vi "EraseRawDataChannels.vi"(7 "error in":errorcluster, 9 "File Limit Size":i64, 10 "TDMS file path in":path) -> (0 "error out":errorcluster, 2 "num chans":i32, 3 "TDMS file path out":path)   [LabVIEW 2012]
uses:
  <vilib>/Platform/storage/lvStorage.llb/_openStorageWithRootAutoDetect.vi
  <vilib>/Platform/storage/lvStorage.llb/xStorage/xStorageSupp/ErrorOut.vi
  <vilib>/Platform/storage/Storage.llb/__loadPropString.vi
  <vilib>/Platform/storage/Storage.llb/__loadPropTime.vi
  <vilib>/Platform/storage/Storage.llb/__loadPropRefList.vi
  <vilib>/Platform/storage/lvStorage.llb/_loadDDT.vi
  <vilib>/Platform/storage/lvStorage.llb/Delete Channel.vi
  <vilib>/Platform/storage/Storage.llb/Get Object Info.vi
  <vilib>/Platform/storage/Storage.llb/__closeStorageFromObject.vi
  <vilib>/ErrorRing/Error Ring.xnode
  <vilib>/Platform/storage/lvStorage.llb/xStorage/Open Data Storage/Open Data Storage.xnode
  <vilib>/Platform/storage/lvStorage.llb/xStorage/Get Properties/Get Properties.xnode
  <vilib>/Platform/storage/lvStorage.llb/xStorage/Close Data Storage/Close Data Storage.xnode
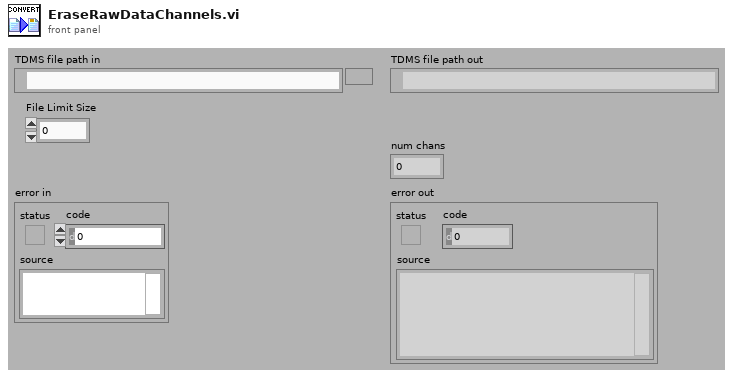
[diagram p1: front panel]
types:
  T1 = enum16{"open", "open or create", "create or replace", "create", "open (read only)"}
  T2 = enum16{"open", "open or create", "create or replace", "create", "open (read-only)"}
  T3 = enum16{"UPDATE", "READ", "QUERY", "CREATE CHILD", "CREATE", "CONNECT", "DISCONNECT"}
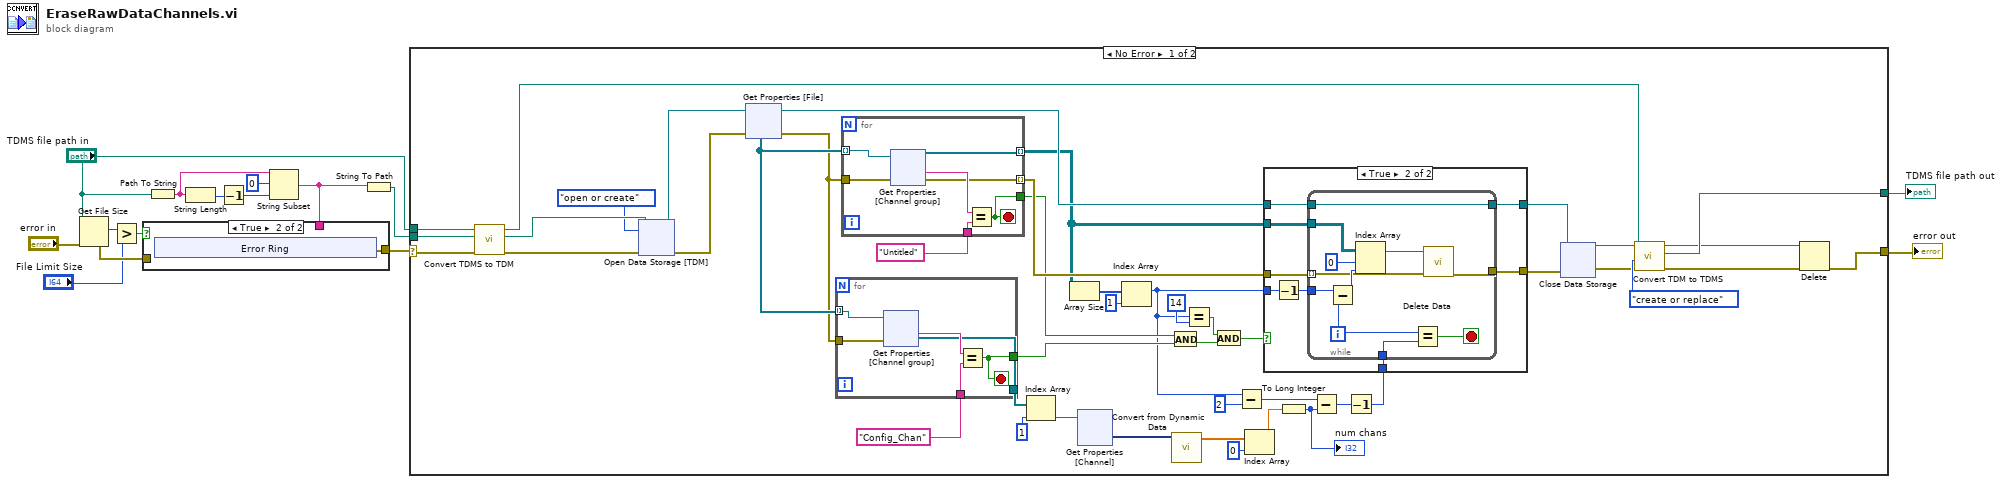
[diagram p0: block diagram]
diagram:
  n1 = Get File Size(file="TDMS file path in", error in="error in") -> (size (in bytes)=w5:i64, 0:w4:errorcluster)  [unwired: 1 out]
  n2 = Greater?(x=w5, y="File Limit Size") -> (0:w6:bool)
  n3 = Path To String(path="TDMS file path in") -> (string=w12:string)
  n4 = String Length(string=w12) -> (length=w13:i32)
  n5 = Decrement(x=w13) -> (x-1=w10:i32)
  n6 = String Subset(string=w12, offset (0)=0, length (rest)=w10) -> (substring=w1:string)
  n7 = case shown="True" w6 {
    tunnel: w4 -> [w16 _]
    tunnel: [w16 w17] -> w3
    tunnel: w1 -> [_ _]
    frame False {
    }
    frame True {
      n8 = xnode "Error Ring"() -> ("error out"=w17:errorcluster)
    }
  }
  n9 = String To Path(string=w1) -> (path=w9:path)
  n10 = case shown="No Error" w3 {
    selector: w3 -> [w57 w193]
    tunnel: [w62 w194] -> w15
    tunnel: [w30 w193] -> w14
    tunnel: "TDMS file path in" -> [w53 w194]
    tunnel: w9 -> [w56 _]
    frame No Error {
      n11 = call <vilib>:"Convert TDMS to TDM.vi"("error in (no error)"=w57, "target file path (*.tdm)"=w56, "source file path (*.tdms)"=w53) -> ("error out"=w60:errorcluster, "target file path (*.tdm) out"=w64:path, "source file path (*.tdms) out"=w52:path)  [unwired: 1 in, 5 out]
      n12 = xnode "Open Data Storage [TDM]"("file path"=w64, "function (open:0)"=T1."open or create" ("fonction (open : 0)"), "error in (no error)"=w60) -> ("storage refnum (file)"=w55:refnum<k20>, "error out"=w54:errorcluster)  [unwired: 2 in, 1 out]
      n13 = xnode "Get Properties [File]"("storage refnum (file)"=w55, "error in"=w54) -> ("storage refnum (file) out"=w36:refnum<k20>, "error out"=w42:errorcluster, "storage refnums (channel group)"=w43:refnum<k20>[])  [unwired: 5 out]
      n14 = for {
        tunnel: w43 -> [w126] mode=indexing
        tunnel: "Config_Chan" ("Group name to delete") -> [w130]
        tunnel: w42 -> [w129]
        tunnel: [w128] -> w38
        tunnel: [w125] -> w51
        stop <- w128 stop-if-true
        n15 = xnode "Get Properties\n[Channel group]"("storage refnum (channel group)"=w126, "error in"=w129) -> ("Name"=w127:string, "storage refnums (channel)"=w125:refnum<k20>[])  [unwired: 3 out]
        n16 = Equal?(x=w127, y=w130) -> (x = y?=w128:bool)
      }
      n17 = for {
        tunnel: w43 -> [w87] mode=indexing
        tunnel: "Untitled" ("Group name to delete") -> [w91]
        tunnel: w42 -> [w90]
        tunnel: [w89] -> w39
        tunnel: [w86] -> w29 mode=indexing
        tunnel: [w85] -> w41 mode=indexing
        stop <- w89 stop-if-true
        n18 = xnode "Get Properties\n[Channel group]"("storage refnum (channel group)"=w87, "error in"=w90) -> ("error out"=w85:errorcluster, "Name"=w88:string, "storage refnums (channel)"=w86:refnum<k20>[])  [unwired: 2 out]
        n19 = Equal?(x=w88, y=w91) -> (x = y?=w89:bool)
      }
      n20 = Index Array(array=w51, index=1) -> (element=w49:refnum<k20>)
      n21 = Array Size(array=w29) -> (size(s)=w33:i32[])
      n22 = xnode "Get Properties\n[Channel]"("storage refnum (channel)"=w49) -> ("Signal"=w48:dynamicdata)  [unwired: 3 in, 4 out]
      n23 = Index Array(array=w33, index=1) -> (element=w20:i32)
      n24 = And(x=w39, y=w38) -> (x .and. y?=w23:bool)
      n25 = call "Convert from Dynamic Data"("Dynamic Data Type"=w48) -> ("Array"=w47:dbl[])  [unwired: 3 in]
      n26 = Equal?(x=w20, y=14) -> (x = y?=w21:bool)
      n27 = And(x=w21, y=w23) -> (x .and. y?=w24:bool)
      n28 = Subtract(x=w20, y=2) -> (x-y=w27:i32)
      n29 = Index Array(array=w47, index=0) -> (element=w45:dbl)
      n30 = To Long Integer(number=w45) -> (32bit integer=w40:i32)
      "num chans" <- w40
      n31 = Subtract(x=w27, y=w40) -> (x-y=w34:i32)
      n32 = Decrement(x=w34) -> (x-1=w26:i32)
      n33 = case shown="True" w24 {
        tunnel: w41 -> [_ w73]
        tunnel: w36 -> [w65 w72]
        tunnel: [w65 w71] -> w35
        tunnel: w29 -> [_ w70]
        tunnel: w20 -> [_ w69]
        tunnel: w26 -> [_ w68]
        tunnel: [_ w66] -> w19
        frame False {
        }
        frame True {
          n34 = Decrement(x=w69) -> (x-1=w67:i32)
          n35 = while {
            tunnel: [w75] -> w66
            tunnel: w73 -> [w77] mode=indexing
            tunnel: w67 -> [w78]
            tunnel: w72 -> [w84]
            tunnel: [w84] -> w71
            tunnel: w68 -> [w83]
            tunnel: w70 -> [w81]
            i -> [w74]
            stop <- w82 stop-if-true
            n36 = Subtract(x=w78, y=w74) -> (x-y=w80:i32)
            n37 = Index Array(array=w81, index (row)=0 ("disabled index (row)"), index (col)=w80) -> (element=w76:refnum<k20>)
            n38 = Equal?(x=w74, y=w83) -> (x = y?=w82:bool)
            n39 = call-poly <vilib>:"Delete Data.vi"("error in (no error)"=w77, "storage refnum (channel)"=w76) -> ("error out"=w75:errorcluster)  [unwired: 5 out]
          }
        }
      }
      n40 = xnode "Close Data Storage"("storage refnum (file)"=w35, "error in (no error)"=w19) -> ("file path"=w32:path, "error out"=w61:errorcluster)
      n41 = call <vilib>:"Convert TDM to TDMS.vi"("error in (no error)"=w61, "target file operation (2:create or replace)"=T2."create or replace", "target file path (*.tdms)"=w52, "source file path (*.tdm)"=w32) -> ("error out"=w31:errorcluster, "target file path (*.tdms) out"=w62:path, "source file path (*.tdm) out"=w25:path)  [unwired: 5 out]
      n42 = Delete(path (use dialog)=w25, error in=w31) -> (error out=w30:errorcluster)  [unwired: 3 in, 2 out]
    }
    frame Error {
    }
  }
  "TDMS file path out" <- w15
  "error out" <- w14
